vi "get http file size.vi"(8 "error in (no error)":errorcluster caption="错误输入（无错误）", 11 "http client 输入":refnum<class "http client.lvclass">) -> (0 "error out":errorcluster caption="错误输出", 2 "文件大小":i64, 3 "http client 输出":refnum<class "http client.lvclass">)   [LabVIEW 2016, in "数据传输系统-02.lvlib" / "update.lvlib" / "http client.lvclass"]
uses:
  http client.lvclass
  http client.lvclass/http client.ctl
  <vilib>/httpClient/LabVIEWHTTPClient.lvlib
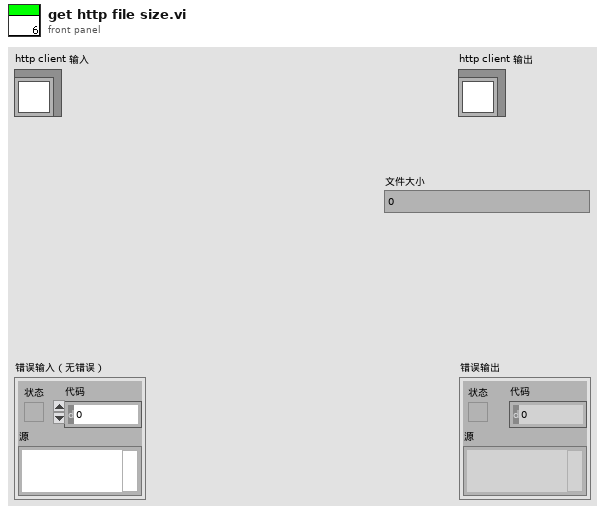
[diagram p1: front panel]
types:
  T1 = typedef "LabVIEWHTTPClient.lvlib/ClientHandle.ctl" = refnum<k1>
  T2 = cluster{"host":string, "port":u16, "user":string, "password":string}
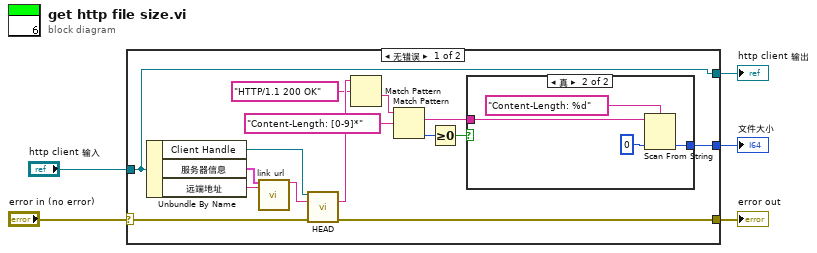
[diagram p0: block diagram]
diagram:
  n1 = case shown="无错误" "error in (no error)" {
    selector: "error in (no error)" -> [w15 w26]
    tunnel: [w14 w26] -> w4
    tunnel: [w20 w25] -> w2
    tunnel: "http client 输入" -> [w20 w25]
    tunnel: [w6 _] -> w1
    frame No Error {
      n2 = Unbundle By Name(w20) -> ("Client Handle"=w19:T1, "服务器信息"=w18:T2, "远端地址"=w17:string)
      n3 = call "link url.vi"("服务器信息"=w18, "远端地址"=w17) -> ("url"=w16:string)  [unwired: 16 in, 1 out]
      n4 = call <vilib>:"HEAD.vi"("client handle"=w19, "url"=w16, "error in (no error)"=w15) -> ("headers"=w13:string, "error out"=w14:errorcluster)  [unwired: 10 in, 1 out]
      n5 = Match Pattern(string=w13, regular expression="HTTP/1.1 200 OK" ("正则表达式")) -> (after substring=w9:string)  [unwired: 1 in, 3 out]
      n6 = Match Pattern(string=w9, regular expression="Content-Length: [0-9]*") -> (match substring=w11:string, offset past match=w8:i32)  [unwired: 1 in, 2 out]
      n7 = Greater Or Equal To 0?(x=w8) -> (x >= 0?=w7:bool)
      n8 = case shown="真" w7 {
        tunnel: w11 -> [_ w22]
        tunnel: [_ w21] -> w6
        frame False {
        }
        frame True {
          n9 = Scan From String(format string="Content-Length: %d", input string=w22, default 1=i64 0 ("default value 1")) -> (output 1=w21:i64)  [unwired: 2 in, 3 out]
        }
      }
    }
    frame Error {
    }
  }
  "error out" <- w4
  "http client 输出" <- w2
  "文件大小" <- w1
